vi "init.vi"(8 "error in (no error)":errorcluster, 11 "Protocol_Generic in":refnum<class "Protocol_Generic.lvclass">) -> (0 "error out":errorcluster, 3 "Protocol_Generic out":refnum<class "Protocol_Generic.lvclass">)   [LabVIEW 2015, in "Protocol_Generic.lvclass"]
uses:
  Protocol_Generic.lvclass
  Protocol_Generic.lvclass/Protocol_Generic.ctl
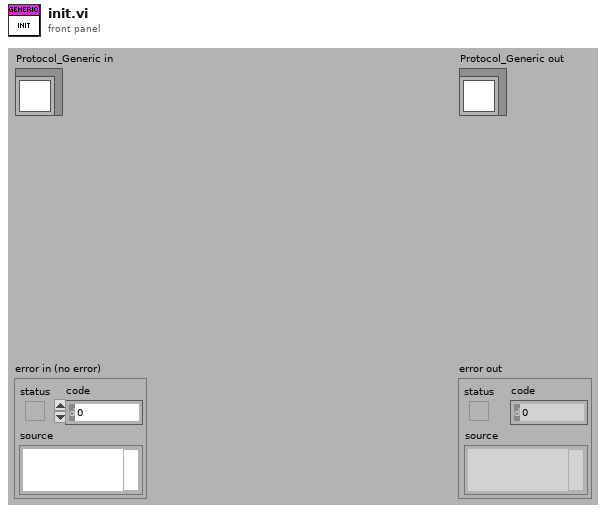
[diagram p1: front panel]
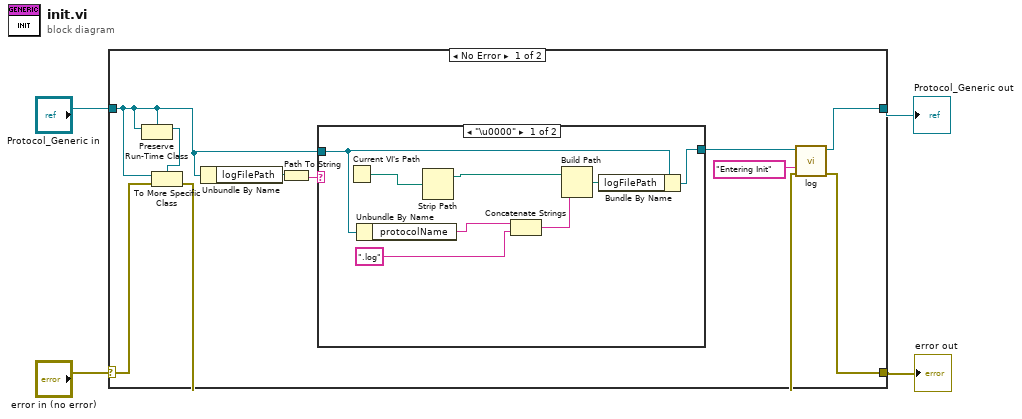
[diagram p0: block diagram]
diagram:
  n1 = case shown="No Error" "error in (no error)" {
    selector: "error in (no error)" -> [w9 w25]
    tunnel: [w14 w25] -> w3
    tunnel: [w5 w24] -> w1
    tunnel: "Protocol_Generic in" -> [w6 w24]
    frame No Error {
      n2 = Preserve Run-Time Class(object in=w6, 2:w6) -> (object out=w7:refnum<class "Protocol_Generic.lvclass">)  [unwired: 1 in, 1 out]
      n3 = To More Specific Class(target class=w7, reference=w6, error in=w9) -> (error out=w8:errorcluster)  [unwired: 1 out]
      n4 = Unbundle By Name(w6) -> ("logFilePath"=w12:path)
      n5 = Path To String(path=w12) -> (string=w11:string)
      n6 = case shown="\"\"" w11 {
        tunnel: w6 -> [w21 w23]
        tunnel: [w22 w23] -> w10
        frame "\u0000" {
          n7 = Current VI's Path() -> (path=w16:path)
          n8 = Unbundle By Name(w21) -> ("protocolName"=w19:string)
          n9 = Strip Path(path=w16) -> (stripped path=w15:path)  [unwired: 1 out]
          n10 = Concatenate Strings(w19, ".log" ("string")) -> (w17:string)
          n11 = Build Path(base path=w15, name or relative path=w17) -> (appended path=w20:path)
          n12 = Bundle By Name(cluster=w21, "logFilePath"=w20) -> (w22:refnum<class "Protocol_Generic.lvclass">)
        }
        frame "actual path", Default {
        }
      }
      n13 = call-dynamic "log.vi"("error in (no error)"=w8, "logLineIn"="Entering Init", "Protocol_Generic in"=w10) -> ("error out"=w14:errorcluster, "Protocol_Generic out"=w5:refnum<class "Protocol_Generic.lvclass">)  [unwired: 7 in]
    }
    frame Error {
    }
  }
  "error out" <- w3
  "Protocol_Generic out" <- w1
